vi "QD_DAQ.vi"(0 "State_and_Data_In":T1, 1 "Max_Queue_Size_In":i32=-1, 2 "Queue_Name_In":string, 5 "Data_In_N":T1[](array[typedef]), 7 "Time_Out_In_ms (-1)":i32, 11 "Error_In":errorcluster, 13 "Queue_Operation":T2=enum."Enqueue") -> (4 "State_and_Data_Out":T1, 15 "Error_Out":errorcluster)   [LabVIEW 2023]
doc: "Used to send the State and event data between loops and VIs"
uses:
  Controls/Queue_Operation_Select.ctl
  Controls/State_and_Data.ctl
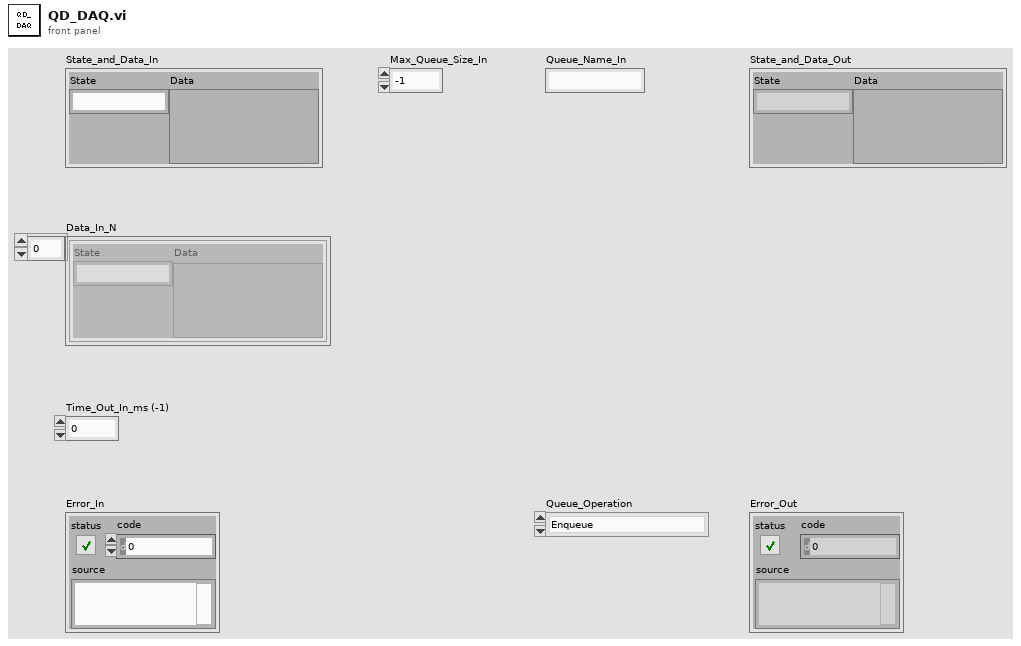
[diagram p1: front panel]
types:
  T1 = typedef "State_and_Data.ctl" = cluster{"State":string, "Data":variant}
  T2 = typedef "Queue_Operation_Select.ctl" = enum16{"Obtain_Queue", "Enqueue", "Enqueue_First", "Enqueue_N", "Lossy_Enqueue", "Preview", "Queue_Status", "Dequeue", "Flush", "Release_Queue"}
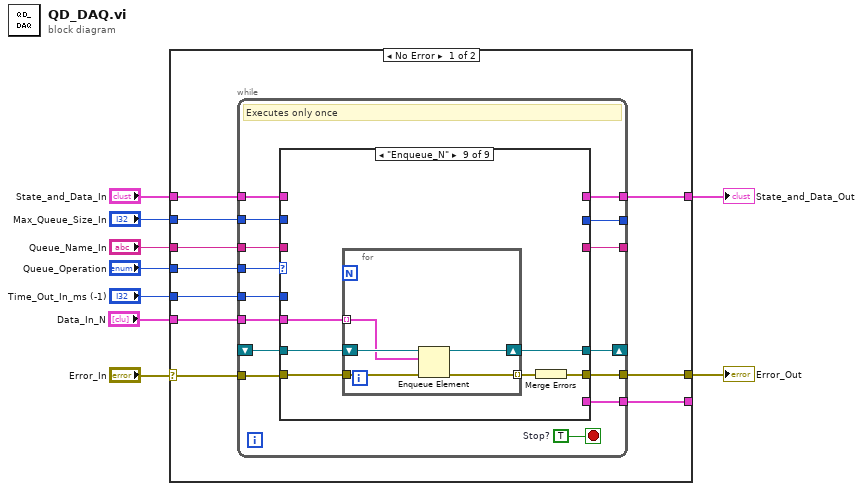
[diagram p0: block diagram]
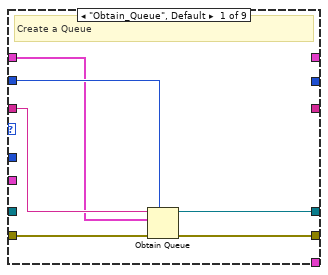
[diagram p2: hidden frame]
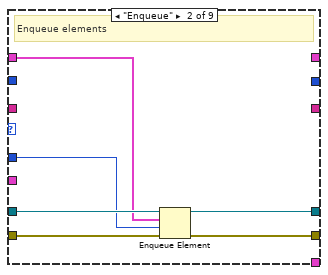
[diagram p3: hidden frame]
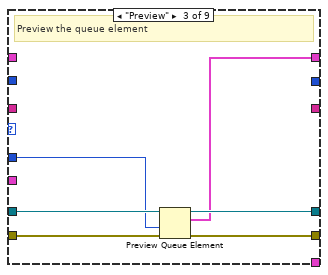
[diagram p4: hidden frame]
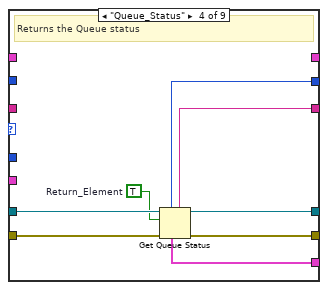
[diagram p5: hidden frame]
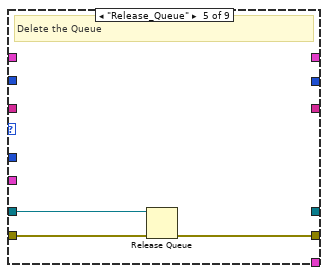
[diagram p6: hidden frame]
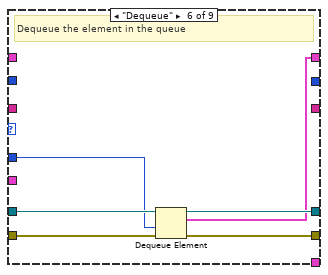
[diagram p7: hidden frame]
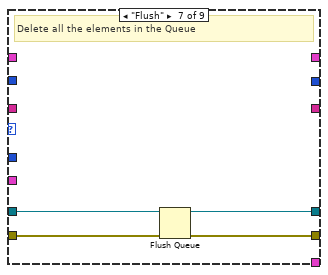
[diagram p8: hidden frame]
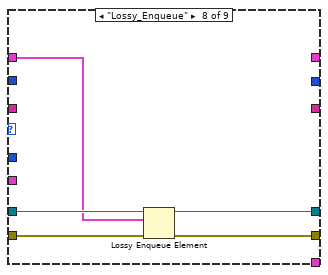
[diagram p9: hidden frame]
diagram:
  n1 = case shown="No Error" "Error_In" {
    selector: "Error_In" -> [w11 w90]
    tunnel: "Max_Queue_Size_In" -> [w19 _]
    tunnel: [w18 w90] -> w8
    tunnel: "State_and_Data_In" -> [w17 _]
    tunnel: "Time_Out_In_ms (-1)" -> [w16 _]
    tunnel: [w15 _] -> w5
    tunnel: "Queue_Operation" -> [w14 _]
    tunnel: "Queue_Name_In" -> [w13 _]
    tunnel: [w12 _] -> _
    tunnel: "Data_In_N" -> [w10 _]
    frame No Error {
      n2 = while {
        tunnel: w19 -> [w34]
        tunnel: w16 -> [w31]
        tunnel: [w29] -> _
        tunnel: w14 -> [w26]
        tunnel: [w24] -> w12
        shift-right: [w27] -> _
        shift-left: _ -> [w22]
        tunnel: w11 -> [w23]
        tunnel: [w33] -> w18
        tunnel: w17 -> [w32]
        tunnel: [w30] -> w15
        tunnel: w13 -> [w25]
        tunnel: [w28] -> _
        tunnel: w10 -> [w20]
        stop <- w21 stop-if-true
        w21 = TRUE  # Stop?
        # "Executes only once"
        n3 = case shown="\"Enqueue_N\"" w26 {
          tunnel: w23 -> [w40 w46 w51 w59 w62 w68 w72 w77 w84]
          tunnel: w25 -> [w38 _ _ _ _ _ _ _ _]
          tunnel: w34 -> [w37 _ _ _ _ _ _ _ _]
          tunnel: [w35 w42 w50 w58 _ w67 w71 w76 w81] -> w27
          tunnel: [w39 w45 w49 w57 w61 w65 w70 w75 w80] -> w33
          tunnel: w22 -> [_ w44 w52 w60 w63 w69 w73 w78 w82]
          tunnel: w32 -> [w36 w43 _ _ _ _ _ w74 _]
          tunnel: w31 -> [_ w41 w48 _ _ w64 _ _ _]
          tunnel: [_ _ w47 _ _ w66 _ _ _] -> w30
          tunnel: [_ _ _ w56 _ _ _ _ _] -> w29
          tunnel: [_ _ _ w55 _ _ _ _ _] -> w28
          tunnel: [_ _ _ w54 _ _ _ _ _] -> w24
          tunnel: w20 -> [_ _ _ _ _ _ _ _ w79]
          frame "Obtain_Queue", Default {
            # "Create a Queue"
            n4 = Obtain Queue(max queue size (-1, unlimited)=w37, name (unnamed)=w38, element data type=w36, error in (no error)=w40) -> (queue out=w35:refnum<queue>, error out=w39:errorcluster)  [unwired: 1 in, 1 out]
          }
          frame "Enqueue" {
            # "Enqueue elements"
            n5 = Enqueue Element(queue=w44, element=w43, timeout in ms (-1)=w41, error in (no error)=w46) -> (queue out=w42:refnum<queue>, error out=w45:errorcluster)  [unwired: 1 out]
          }
          frame "Preview" {
            # "Preview the queue element"
            n6 = Preview Queue Element(queue=w52, timeout in ms (-1)=w48, error in (no error)=w51) -> (queue out=w50:refnum<queue>, element=w47:T1, error out=w49:errorcluster)  [unwired: 1 out]
          }
          frame "Queue_Status" {
            w53 = TRUE  # Return_Element
            # "Returns the Queue status"
            n7 = Get Queue Status(queue=w60, return elements? (F)=w53, error in (no error)=w59) -> (queue out=w58:refnum<queue>, queue name=w55:string, max queue size=w56:i32, error out=w57:errorcluster, elements=w54:T1[])  [unwired: 3 out]
          }
          frame "Release_Queue" {
            # "Delete the Queue"
            n8 = Release Queue(queue=w63, error in (no error)=w62) -> (error out=w61:errorcluster)  [unwired: 1 in, 2 out]
          }
          frame "Dequeue" {
            # "Dequeue the element in the queue"
            n9 = Dequeue Element(queue=w69, timeout in ms (-1)=w64, error in (no error)=w68) -> (queue out=w67:refnum<queue>, element=w66:T1, error out=w65:errorcluster)  [unwired: 1 out]
          }
          frame "Flush" {
            # "Delete all the elements in the Queue"
            n10 = Flush Queue(queue=w73, error in (no error)=w72) -> (queue out=w71:refnum<queue>, error out=w70:errorcluster)  [unwired: 1 out]
          }
          frame "Lossy_Enqueue" {
            n11 = Lossy Enqueue Element(queue=w78, element=w74, error in (no error)=w77) -> (queue out=w76:refnum<queue>, error out=w75:errorcluster)  [unwired: 2 out]
          }
          frame "Enqueue_N" {
            n12 = for {
              tunnel: w84 -> [w89]
              tunnel: [w88] -> w83 mode=indexing
              shift-right: [w86] -> w81
              shift-left: w82 -> [w87]
              tunnel: w79 -> [w85] mode=indexing
              n13 = Enqueue Element(queue=w87, element=w85, error in (no error)=w89) -> (queue out=w86:refnum<queue>, error out=w88:errorcluster)  [unwired: 1 in, 1 out]
            }
            n14 = Merge Errors(w83) -> (w80:errorcluster)
          }
        }
      }
    }
    frame Error {
    }
  }
  "Error_Out" <- w8
  "State_and_Data_Out" <- w5
